vi "Read inventory.vi"(8 "error in (no error)":errorcluster, 11 "User Interface in":refnum<class "User Interface.lvclass">) -> (0 "error out":errorcluster, 2 "inventory":cluster{"String":string, "value":u32, bool}[][](array[cluster]), 3 "User Interface out":refnum<class "User Interface.lvclass">)   [LabVIEW 2020, in "User Interface.lvlib" / "User Interface.lvclass"]
uses:
  User Interface.lvclass
  <vilib>/Utility/config.llb/Read Key (U32).vi
  <vilib>/Utility/config.llb/NI_LVConfig.lvlib
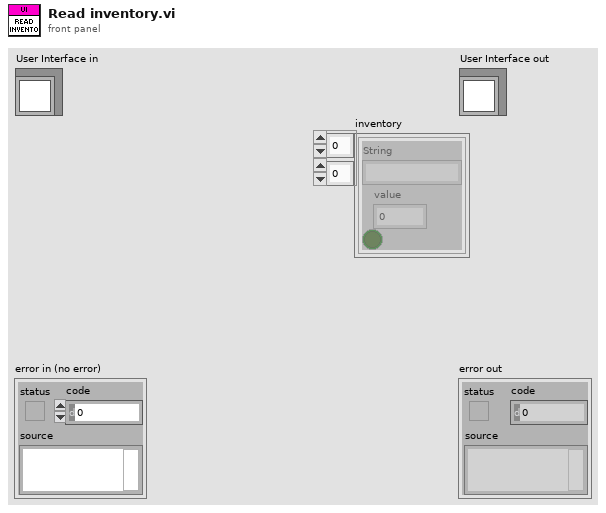
[diagram p1: front panel]
types:
  T1 = typedef "NI_LVConfig.lvlib/Config Data RefNum.ctl" = refnum<k1>
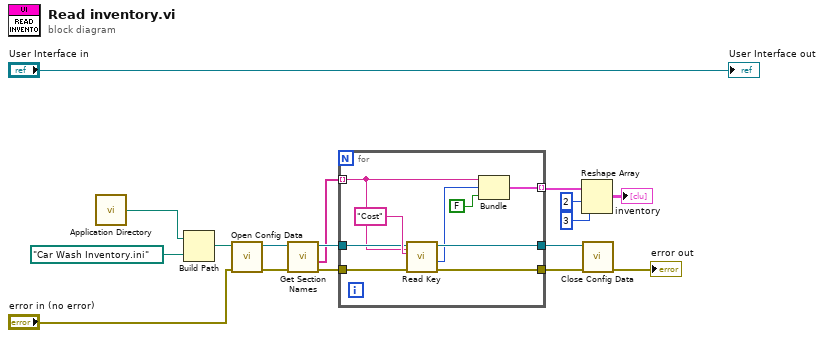
[diagram p0: block diagram]
diagram:
  n1 = call <vilib>:"Application Directory.vi"() -> ("Application Directory"=w17:path)
  n2 = Build Path(base path=w17, name or relative path=path "Car Wash Inventory.ini") -> (appended path=w14:path)
  n3 = call <vilib>:"Open Config Data.vi"("error in (no error)"="error in (no error)", "configuration file path"=w14) -> ("error out"=w15:errorcluster, "refnum"=w9:T1)  [unwired: 7 in, 1 out]
  n4 = call <vilib>:"Get Section Names.vi"("error in (no error)"=w15, "refnum"=w9) -> ("error out"=w13:errorcluster, "section names"=w8:string[], "refnum out"=w10:T1)  [unwired: 7 in]
  n5 = for {
    tunnel: w13 -> [w26]
    tunnel: [w25] -> w12
    tunnel: [w23] -> w11
    tunnel: w10 -> [w22]
    tunnel: [w19] -> _ mode=indexing
    tunnel: w8 -> [w19] mode=indexing
    tunnel: [w20] -> w7 mode=indexing
    n6 = call-poly <vilib>:"Read Key.vi"("section"=w19, "error in (no error)"=w26, "key"="Cost", "refnum"=w22) -> ("error out"=w25:errorcluster, "value"=w21:u32, "refnum out"=w23:T1)  [unwired: 4 in, 1 out]
    n7 = Bundle("String"=w19, "value"=w21, FALSE) -> (w20:cluster{"String":string, "value":u32, bool})  [unwired: 1 in]
  }
  n8 = Reshape Array(w7, 2 ("dimension size"), 3 ("dimension size")) -> (→"inventory":cluster{"String":string, "value":u32, bool}[][])
  n9 = call <vilib>:"Close Config Data.vi"("error in (no error)"=w12, "refnum"=w11) -> ("error out"=→"error out":errorcluster)  [unwired: 8 in, 1 out]
  "User Interface out" <- "User Interface in"
